vi "SaveP0(air).vi"(7 "error in (no error)":errorcluster, 10 "OSA Setting":T1={"CENTER(nm)"="850", "SPAN(nm)"="700", "RESOLUTION(nm)"="10", "SAMPLING(point)"="1001", "NEARBY AVG(point)"=50} {"NEARBY AVG(point)" min=0 max=300}) -> (0 "error out":errorcluster, 1 "Power":dbl[](array[numeric])=[0.0, 0.0, 0.0, 0.0, 0.0, 0.0, 0.0, 0.0, 0.0, 0.0, 0.0, 0.0, 0.0, 0.0, 0.0, 0.0, 0.0, 0.0, 0.0, 0.0, 0.0, 0.0, 0.0, 0.0, 0.0, 0.0, 0.0, 0.0, 0.0, 0.0, 0.0, 0.0, 0.0, 0.0, 0.0, 0.0, 0.0, 0.0, 0.0, 0.0, 0.0, 0.0, 0.0, 0.0, 0.0, 0.0, 0.0, 0.0, 0.0, 0.0, 0.0, 0.0, 0.0, 0.0, 0.0, 0.0, 0.0, 0.0, 0.0, 0.0, 0.0, 0.0, 0.0, 0.0, 0.0, 0.0, 0.0, 0.0, 0.0, 0.0, 0.0, 0.0, 0.0, 0.0, 0.0, 0.0, 0.0, 0.0, 0.0, 0.0, 0.0, 0.0, 0.0, 0.0, 0.0, 0.0, 0.0, 0.0, 0.0, 0.0, 0.0, 0.0, 0.0, 0.0, 0.0, 0.0, 0.0, 0.0, 0.0, 0.0, 0.0, 0.0, 0.0, 0.0, 0.0, 0.0, 0.0, 0.0, 0.0, 0.0, 0.0, 0.0, 0.0, 0.0, 0.0, 4.604e-06, 4.226e-06, 3.975e-06, 3.889e-06, 3.711e-06, 3.198e-06, 3.37e-06, 3.06e-06, 2.761e-06, 2.723e-06, 2.421e-06, 2.456e-06, 2.236e-06, 2.262e-06, 1.844e-06, 1.89e-06, 1.693e-06, 1.559e-06, 1.574e-06, 1.384e-06, 1.509e-06, 1.223e-06, 1.135e-06, 1.015e-06, 1.019e-06, 1.063e-06, 1.12e-06, 1.008e-06, 9.191e-07, 8.066e-07, 9.947e-07, 8.717e-07, 7.15e-07, 3.58e-07, 6.616e-07, 2.625e-07, 6.819e-07, 5.007e-07, 5.837e-07, 3.041e-07, 3.955e-07, 2.946e-07, 2.786e-07, 4.332e-07, 3.147e-07, 4.411e-07, 3.222e-07, 5.534e-07, 4.934e-07, 3.092e-07, 4.549e-07, 3.537e-07, 5.085e-07, 5.492e-07, 3.821e-07, 1.417e-07, 1.836e-07, 4.04e-07, 3.374e-07, 2.833e-07, 4.353e-07, 4.327e-07, 4.769e-07, 2.7e-07, 4.071e-07, 5.302e-07, 2.895e-07, 4.622e-07, 2.297e-07, 3.785e-07, 5.313e-07, 4.222e-07, 4.187e-07, 4.765e-07, 2.779e-07, 4.899e-07, 3.572e-07, 4.825e-07, 4.047e-07, 2.323e-07, 4.424e-07, 3.741e-07, 3.112e-07, 3.263e-07, 5.85e-07, 3.807e-07, 4.832e-07, 3.282e-07, 5.253e-07, 5.721e-07, 3.284e-07, 5.965e-07, 5.382e-07, 6.57e-07, 6.003e-07, 5.373e-07, 2.205e-07, 2.197e-07, 4.956e-07, 5.32e-07, 6.087e-07, 5.617e-07, 3.005e-07, 2.958e-07, 4.149e-07, 5.546e-07, 4.977e-07, 5.231e-07, 4.014e-07, 5.628e-07, 4.117e-07, 5.73e-07, 5.151e-07, 5.486e-07, 4.807e-07, 4.761e-07, 7.077e-07, 4.602e-07, 6.771e-07, 6.071e-07, 6.961e-07, 6.177e-07, 4.859e-07, 7.841e-07, 6.593e-07, 7.061e-07, 7.447e-07, 7.425e-07, 6.849e-07, 8.248e-07, 7.253e-07, 6.385e-07, 5.973e-07, 7.055e-07, 9.005e-07, 6.834e-07, 7.497e-07, 7.568e-07, 7.572e-07, 6.431e-07, 7.918e-07, 7.715e-07, 8.923e-07, 9.456e-07, 8.613e-07, 7.157e-07, 8.648e-07, 9.133e-07, 8.563e-07, 8.122e-07, 8.679e-07, 9.508e-07, 8.59e-07, 8.475e-07, 9.19e-07, 7.877e-07, 8.525e-07, 9.693e-07, 9.565e-07, 9.64e-07, 9.516e-07, 9.918e-07, 9.921e-07, 9.24e-07, 9.257e-07, 9.966e-07, 1.017e-06, 1.008e-06, 1.046e-06, 9.957e-07, 1.008e-06, 9.996e-07, 1.162e-06, 1.04e-06, 1.153e-06, 1.19e-06, 1.151e-06, 1.036e-06, 1.183e-06, 1.253e-06, 1.113e-06, 1.186e-06, 1.175e-06, 1.156e-06, 1.232e-06, 1.183e-06, 1.203e-06, 1.293e-06, 1.303e-06, 1.256e-06, 1.223e-06, 1.332e-06, 1.313e-06, 1.354e-06, 1.179e-06, 1.332e-06, 1.405e-06, 1.37e-06, 1.48e-06, 1.411e-06, 5.115e-06, 5.245e-06, 5.299e-06, 5.328e-06, 5.298e-06, 5.443e-06, 5.469e-06, 5.779e-06, 5.733e-06, 5.651e-06, 5.691e-06, 5.718e-06, 5.813e-06, 5.937e-06, 6.012e-06, 6e-06, 6.008e-06, 6.105e-06, 6.046e-06, 6.014e-06, 6.085e-06, 5.952e-06, 5.963e-06, 5.892e-06, 5.992e-06, 5.988e-06, 6.057e-06, 6.126e-06, 6.143e-06, 6.149e-06, 6.281e-06, 6.341e-06, 6.312e-06, 6.395e-06, 6.426e-06, 6.446e-06, 6.497e-06, 6.625e-06, 6.554e-06, 6.759e-06, 6.725e-06, 6.679e-06, 6.767e-06, 6.895e-06, 6.907e-06, 7.068e-06, 7.076e-06, 7.064e-06, 7.228e-06, 7.205e-06, 7.393e-06, 7.487e-06, 7.401e-06, 7.538e-06, 7.579e-06, 7.667e-06, 7.736e-06, 7.748e-06, 7.781e-06, 8.029e-06, 8.021e-06, 8.011e-06, 8.174e-06, 8.176e-06, 8.232e-06, 8.256e-06, 8.341e-06, 8.428e-06, 8.462e-06, 8.486e-06, 8.625e-06, 8.696e-06, 8.716e-06, 8.832e-06, 8.847e-06, 8.972e-06, 9.087e-06, 9.166e-06, 9.088e-06, 9.273e-06, 9.281e-06, 9.285e-06, 9.345e-06, 9.43e-06, 9.467e-06, 9.631e-06, 9.643e-06, 9.694e-06, 9.801e-06, 9.802e-06, 1e-05, 9.924e-06, 1.001e-05, 1.012e-05, 1.013e-05, 1.024e-05, 1.033e-05, 1.037e-05, 1.046e-05, 1.042e-05, 1.058e-05, 1.061e-05, 1.073e-05, 1.073e-05, 1.09e-05, 1.086e-05, 1.101e-05, 1.11e-05, 1.115e-05, 1.127e-05, 1.109e-05, 1.124e-05, 1.132e-05, 1.137e-05, 1.143e-05, 1.147e-05, 1.15e-05, 1.159e-05, 1.156e-05, 1.154e-05, 1.174e-05, 1.176e-05, 1.188e-05, 1.155e-05, 1.193e-05, 1.21e-05, 1.194e-05, 1.214e-05, 1.205e-05, 1.212e-05, 1.215e-05, 1.2e-05, 1.222e-05, 1.216e-05, 1.215e-05, 1.239e-05, 1.241e-05, 1.222e-05, 1.257e-05, 1.28e-05, 1.255e-05, 1.262e-05, 1.293e-05, 1.305e-05, 1.312e-05, 1.314e-05, 1.337e-05, 1.32e-05, 1.324e-05, 1.344e-05, 1.352e-05, 1.352e-05, 1.347e-05, 1.366e-05, 1.388e-05, 1.382e-05, 1.386e-05, 1.397e-05, 1.409e-05, 1.393e-05, 1.372e-05, 1.392e-05, 1.418e-05, 1.404e-05, 1.434e-05, 1.43e-05, 1.419e-05, 1.433e-05, 1.438e-05, 1.427e-05, 1.45e-05, 1.459e-05, 1.465e-05, 1.466e-05, 1.471e-05, 1.49e-05, 1.494e-05, 1.504e-05, 1.498e-05, 1.497e-05, 1.515e-05, 1.507e-05, 1.512e-05, 1.525e-05, 1.498e-05, 1.523e-05, 1.529e-05, 1.536e-05, 1.523e-05, 1.567e-05, 1.547e-05, 1.549e-05, 1.529e-05, 1.539e-05, 1.538e-05, 1.556e-05, 1.554e-05, 1.57e-05, 1.585e-05, 1.594e-05, 1.594e-05, 1.58e-05, 1.582e-05, 1.631e-05, 1.616e-05, 1.631e-05, 1.638e-05, 1.631e-05, 1.648e-05, 1.648e-05, 1.653e-05, 1.638e-05, 1.649e-05, 1.655e-05, 1.657e-05, 1.646e-05, 1.649e-05, 1.621e-05, 1.657e-05, 1.659e-05, 1.657e-05, 1.637e-05, 1.66e-05, 1.662e-05, 1.661e-05, 1.678e-05, 1.665e-05, 1.702e-05, 1.665e-05, 1.717e-05, 1.718e-05, 1.699e-05, 1.709e-05, 1.722e-05, 1.729e-05, 1.737e-05, 1.743e-05, 1.732e-05, 1.747e-05, 1.747e-05, 1.736e-05, 1.725e-05, 1.74e-05, 1.717e-05, 1.745e-05, 1.737e-05, 1.733e-05, 1.738e-05, 1.742e-05, 1.737e-05, 1.749e-05, 1.761e-05, 1.749e-05, 1.747e-05, 1.736e-05, 1.748e-05, 1.758e-05, 2.446e-05, 2.448e-05, 2.45e-05, 2.477e-05, 2.464e-05, 2.468e-05, 2.473e-05, 2.475e-05, 2.478e-05, 2.503e-05, 2.484e-05, 2.503e-05, 2.493e-05, 2.5e-05, 2.497e-05, 2.511e-05, 2.512e-05, 2.51e-05, 2.536e-05, 2.521e-05, 2.531e-05, 2.536e-05, 2.549e-05, 2.546e-05, 2.55e-05, 2.546e-05, 2.549e-05, 2.566e-05, 2.56e-05, 2.56e-05, 2.552e-05, 2.578e-05, 2.577e-05, 2.586e-05, 2.576e-05, 2.577e-05, 2.584e-05, 2.577e-05, 2.599e-05, 2.589e-05, 2.591e-05, 2.623e-05, 2.609e-05, 2.613e-05, 2.618e-05, 2.63e-05, 2.609e-05, 2.623e-05, 2.627e-05, 2.647e-05, 2.646e-05, 2.654e-05, 2.65e-05, 2.648e-05, 2.648e-05, 2.647e-05, 2.694e-05, 2.651e-05, 2.671e-05, 2.675e-05, 2.69e-05, 2.683e-05, 2.71e-05, 2.693e-05, 2.693e-05, 2.713e-05, 2.707e-05, 2.724e-05, 2.722e-05, 2.738e-05, 2.734e-05, 2.743e-05, 2.745e-05, 2.722e-05, 2.762e-05, 2.765e-05, 2.769e-05, 2.782e-05, 2.771e-05, 2.793e-05, 2.806e-05, 2.807e-05, 2.823e-05, 2.838e-05, 2.836e-05, 2.841e-05, 2.855e-05, 2.865e-05, 2.88e-05, 2.891e-05, 2.896e-05, 2.898e-05, 2.9e-05, 2.906e-05, 2.905e-05, 2.913e-05, 2.909e-05, 2.904e-05, 2.942e-05, 2.918e-05, 2.936e-05, 2.948e-05, 2.952e-05, 2.955e-05, 2.951e-05, 2.958e-05, 2.963e-05, 2.99e-05, 2.989e-05, 2.997e-05, 3.012e-05, 3.006e-05, 3.009e-05, 3.016e-05, 3.039e-05, 3.04e-05, 3.053e-05, 3.051e-05, 3.052e-05, 3.074e-05, 3.064e-05, 3.06e-05, 3.082e-05, 3.086e-05, 3.073e-05, 3.095e-05, 3.096e-05, 3.094e-05, 3.092e-05, 3.109e-05, 3.099e-05, 3.098e-05, 3.107e-05, 3.114e-05, 3.131e-05, 3.129e-05, 3.129e-05, 3.146e-05, 3.147e-05, 3.147e-05, 3.159e-05, 3.18e-05, 3.17e-05, 3.166e-05, 3.191e-05, 3.184e-05, 3.196e-05, 3.218e-05, 3.219e-05, 3.233e-05, 3.23e-05, 3.25e-05, 3.265e-05, 3.258e-05, 3.264e-05, 3.268e-05, 3.27e-05, 3.276e-05, 3.282e-05, 3.287e-05, 3.288e-05, 3.285e-05, 3.298e-05, 3.314e-05, 3.324e-05, 3.337e-05, 3.338e-05, 3.336e-05, 3.329e-05, 3.344e-05, 3.356e-05, 3.375e-05, 3.382e-05, 3.376e-05, 3.378e-05, 3.373e-05, 3.391e-05, 3.4e-05, 3.405e-05, 3.417e-05, 3.42e-05, 3.443e-05, 3.431e-05, 3.435e-05, 3.445e-05, 3.431e-05, 3.446e-05, 3.448e-05, 3.449e-05, 3.467e-05, 3.455e-05, 3.47e-05, 3.483e-05, 3.498e-05, 3.476e-05, 3.492e-05, 3.492e-05, 3.502e-05, 3.515e-05, 3.522e-05, 3.538e-05, 3.537e-05, 3.537e-05, 3.553e-05, 3.55e-05, 3.56e-05, 3.57e-05, 3.583e-05, 3.578e-05, 3.592e-05, 3.603e-05, 3.601e-05, 3.605e-05, 3.61e-05, 3.615e-05, 3.627e-05, 3.638e-05, 3.621e-05, 3.619e-05, 3.639e-05, 3.632e-05, 3.651e-05, 3.647e-05, 3.671e-05, 3.668e-05, 3.675e-05, 3.66e-05, 3.677e-05, 3.664e-05, 3.686e-05, 3.655e-05, 3.676e-05, 3.666e-05, 3.667e-05, 3.667e-05, 3.661e-05, 3.66e-05, 3.674e-05, 3.673e-05, 3.659e-05, 3.68e-05, 3.678e-05, 3.684e-05, 3.678e-05, 3.672e-05, 3.669e-05, 3.672e-05, 3.664e-05, 3.661e-05, 3.665e-05, 3.68e-05, 3.669e-05, 3.679e-05, 3.678e-05, 3.713e-05, 3.693e-05, 3.724e-05, 3.724e-05, 3.73e-05, 3.738e-05, 3.742e-05, 3.764e-05, 3.771e-05, 3.766e-05, 3.786e-05, 3.787e-05, 3.778e-05, 3.779e-05, 3.771e-05, 3.767e-05, 3.755e-05, 3.742e-05, 3.749e-05, 3.756e-05, 3.756e-05, 3.759e-05, 3.748e-05, 3.769e-05, 3.778e-05, 3.785e-05, 3.787e-05, 3.812e-05, 3.799e-05, 3.811e-05, 3.822e-05, 3.832e-05, 3.828e-05, 3.838e-05, 3.87e-05, 3.863e-05, 3.879e-05, 3.871e-05, 3.877e-05, 3.883e-05, 3.872e-05, 3.891e-05, 3.877e-05, 3.9e-05, 3.898e-05, 3.905e-05, 3.885e-05, 3.892e-05, 3.89e-05, 3.901e-05, 3.879e-05, 3.89e-05, 3.885e-05, 3.891e-05, 3.895e-05, 3.89e-05, 3.891e-05, 3.883e-05, 3.875e-05, 3.872e-05, 3.896e-05, 3.883e-05, 3.888e-05, 3.9e-05, 3.899e-05, 3.914e-05, 3.913e-05, 3.923e-05, 3.929e-05, 3.932e-05, 3.936e-05, 3.914e-05, 3.924e-05, 3.95e-05, 3.932e-05, 3.929e-05, 3.931e-05, 3.938e-05, 3.918e-05, 3.9280000000000003e-05, 3.925e-05, 3.936e-05, 3.947e-05, 3.912e-05, 3.931e-05, 3.945e-05, 3.94e-05, 3.941e-05, 3.94e-05, 3.913e-05, 3.903e-05, 3.915e-05, 3.908e-05, 3.912e-05, 3.903e-05, 3.89e-05, 3.898e-05, 3.885e-05, 3.881e-05, 3.883e-05, 3.879e-05, 3.886e-05, 3.904e-05, 3.903e-05, 3.891e-05, 3.871e-05, 3.868e-05, 3.847e-05, 3.858e-05, 3.857e-05, 3.846e-05, 3.852e-05, 3.857e-05, 3.871e-05, 3.873e-05, 3.859e-05, 3.87e-05, 3.88e-05, 3.862e-05, 3.851e-05, 3.855e-05, 3.837e-05, 3.839e-05, 3.831e-05, 3.84e-05, 3.833e-05, 3.844e-05, 3.835e-05, 3.838e-05, 3.837e-05, 3.84e-05, 3.845e-05, 3.835e-05, 3.841e-05, 3.82e-05, 3.82e-05, 3.805e-05, 3.808e-05, 3.801e-05, 3.788e-05, 3.796e-05, 3.797e-05, 3.778e-05, 3.795e-05, 3.768e-05, 3.771e-05, 3.783e-05, 3.767e-05, 3.754e-05, 3.754e-05, 3.761e-05, 3.76e-05, 3.774e-05, 3.765e-05, 3.757e-05, 3.777e-05, 3.755e-05, 3.753e-05, 3.754e-05, 3.758e-05, 3.758e-05, 3.771e-05, 3.766e-05, 3.766e-05, 3.781e-05, 3.785e-05, 3.791e-05, 3.799e-05, 3.795e-05, 3.794e-05, 3.808e-05, 3.79e-05, 3.809e-05, 3.798e-05, 3.794e-05], 3 "Wavelength":dbl[](array[numeric])=[250.0, 250.7, 251.4, 252.1, 252.8, 253.5, 254.2, 254.9, 255.6, 256.3, 257.0, 257.7, 258.4, 259.1, 259.8, 260.5, 261.2, 261.9, 262.6, 263.3, 264.0, 264.7, 265.4, 266.1, 266.8, 267.5, 268.2, 268.9, 269.6, 270.3, 271.0, 271.7, 272.4, 273.1, 273.8, 274.5, 275.2, 275.9, 276.6, 277.3, 278.0, 278.7, 279.4, 280.1, 280.8, 281.5, 282.2, 282.9, 283.6, 284.3, 285.0, 285.7, 286.4, 287.1, 287.8, 288.5, 289.2, 289.9, 290.6, 291.3, 292.0, 292.7, 293.4, 294.1, 294.8, 295.5, 296.2, 296.9, 297.6, 298.3, 299.0, 299.7, 300.4, 301.1, 301.8, 302.5, 303.2, 303.9, 304.6, 305.3, 306.0, 306.7, 307.4, 308.1, 308.8, 309.5, 310.2, 310.9, 311.6, 312.3, 313.0, 313.7, 314.4, 315.1, 315.8, 316.5, 317.2, 317.9, 318.6, 319.3, 320.0, 320.7, 321.4, 322.1, 322.8, 323.5, 324.2, 324.9, 325.6, 326.3, 327.0, 327.7, 328.4, 329.1, 329.8, 330.5, 331.2, 331.9, 332.6, 333.3, 334.0, 334.7, 335.4, 336.1, 336.8, 337.5, 338.2, 338.9, 339.6, 340.3, 341.0, 341.7, 342.4, 343.1, 343.8, 344.5, 345.2, 345.9, 346.6, 347.3, 348.0, 348.7, 349.4, 350.1, 350.8, 351.5, 352.2, 352.9, 353.6, 354.3, 355.0, 355.7, 356.4, 357.1, 357.8, 358.5, 359.2, 359.9, 360.6, 361.3, 362.0, 362.7, 363.4, 364.1, 364.8, 365.5, 366.2, 366.9, 367.6, 368.3, 369.0, 369.7, 370.4, 371.1, 371.8, 372.5, 373.2, 373.9, 374.6, 375.3, 376.0, 376.7, 377.4, 378.1, 378.8, 379.5, 380.2, 380.9, 381.6, 382.3, 383.0, 383.7, 384.4, 385.1, 385.8, 386.5, 387.2, 387.9, 388.6, 389.3, 390.0, 390.7, 391.4, 392.1, 392.8, 393.5, 394.2, 394.9, 395.6, 396.3, 397.0, 397.7, 398.4, 399.1, 399.8, 400.5, 401.2, 401.9, 402.6, 403.3, 404.0, 404.7, 405.4, 406.1, 406.8, 407.5, 408.2, 408.9, 409.6, 410.3, 411.0, 411.7, 412.4, 413.1, 413.8, 414.5, 415.2, 415.9, 416.6, 417.3, 418.0, 418.7, 419.4, 420.1, 420.8, 421.5, 422.2, 422.9, 423.6, 424.3, 425.0, 425.7, 426.4, 427.1, 427.8, 428.5, 429.2, 429.9, 430.6, 431.3, 432.0, 432.7, 433.4, 434.1, 434.8, 435.5, 436.2, 436.9, 437.6, 438.3, 439.0, 439.7, 440.4, 441.1, 441.8, 442.5, 443.2, 443.9, 444.6, 445.3, 446.0, 446.7, 447.4, 448.1, 448.8, 449.5, 450.2, 450.9, 451.6, 452.3, 453.0, 453.7, 454.4, 455.1, 455.8, 456.5, 457.2, 457.9, 458.6, 459.3, 460.0, 460.7, 461.4, 462.1, 462.8, 463.5, 464.2, 464.9, 465.6, 466.3, 467.0, 467.7, 468.4, 469.1, 469.8, 470.5, 471.2, 471.9, 472.6, 473.3, 474.0, 474.7, 475.4, 476.1, 476.8, 477.5, 478.2, 478.9, 479.6, 480.3, 481.0, 481.7, 482.4, 483.1, 483.8, 484.5, 485.2, 485.9, 486.6, 487.3, 488.0, 488.7, 489.4, 490.1, 490.8, 491.5, 492.2, 492.9, 493.6, 494.3, 495.0, 495.7, 496.4, 497.1, 497.8, 498.5, 499.2, 499.9, 500.6, 501.3, 502.0, 502.7, 503.4, 504.1, 504.8, 505.5, 506.2, 506.9, 507.6, 508.3, 509.0, 509.7, 510.4, 511.1, 511.8, 512.5, 513.2, 513.9, 514.6, 515.3, 516.0, 516.7, 517.4, 518.1, 518.8, 519.5, 520.2, 520.9, 521.6, 522.3, 523.0, 523.7, 524.4, 525.1, 525.8, 526.5, 527.2, 527.9, 528.6, 529.3, 530.0, 530.7, 531.4, 532.1, 532.8, 533.5, 534.2, 534.9, 535.6, 536.3, 537.0, 537.7, 538.4, 539.1, 539.8, 540.5, 541.2, 541.9, 542.6, 543.3, 544.0, 544.7, 545.4, 546.1, 546.8, 547.5, 548.2, 548.9, 549.6, 550.3, 551.0, 551.7, 552.4, 553.1, 553.8, 554.5, 555.2, 555.9, 556.6, 557.3, 558.0, 558.7, 559.4, 560.1, 560.8, 561.5, 562.2, 562.9, 563.6, 564.3, 565.0, 565.7, 566.4, 567.1, 567.8, 568.5, 569.2, 569.9, 570.6, 571.3, 572.0, 572.7, 573.4, 574.1, 574.8, 575.5, 576.2, 576.9, 577.6, 578.3, 579.0, 579.7, 580.4, 581.1, 581.8, 582.5, 583.2, 583.9, 584.6, 585.3, 586.0, 586.7, 587.4, 588.1, 588.8, 589.5, 590.2, 590.9, 591.6, 592.3, 593.0, 593.7, 594.4, 595.1, 595.8, 596.5, 597.2, 597.9, 598.6, 599.3, 600.0, 600.7, 601.4, 602.1, 602.8, 603.5, 604.2, 604.9, 605.6, 606.3, 607.0, 607.7, 608.4, 609.1, 609.8, 610.5, 611.2, 611.9, 612.6, 613.3, 614.0, 614.7, 615.4, 616.1, 616.8, 617.5, 618.2, 618.9, 619.6, 620.3, 621.0, 621.7, 622.4, 623.1, 623.8, 624.5, 625.2, 625.9, 626.6, 627.3, 628.0, 628.7, 629.4, 630.1, 630.8, 631.5, 632.2, 632.9, 633.6, 634.3, 635.0, 635.7, 636.4, 637.1, 637.8, 638.5, 639.2, 639.9, 640.6, 641.3, 642.0, 642.7, 643.4, 644.1, 644.8, 645.5, 646.2, 646.9, 647.6, 648.3, 649.0, 649.7, 650.4, 651.1, 651.8, 652.5, 653.2, 653.9, 654.6, 655.3, 656.0, 656.7, 657.4, 658.1, 658.8, 659.5, 660.2, 660.9, 661.6, 662.3, 663.0, 663.7, 664.4, 665.1, 665.8, 666.5, 667.2, 667.9, 668.6, 669.3, 670.0, 670.7, 671.4, 672.1, 672.8, 673.5, 674.2, 674.9, 675.6, 676.3, 677.0, 677.7, 678.4, 679.1, 679.8, 680.5, 681.2, 681.9, 682.6, 683.3, 684.0, 684.7, 685.4, 686.1, 686.8, 687.5, 688.2, 688.9, 689.6, 690.3, 691.0, 691.7, 692.4, 693.1, 693.8, 694.5, 695.2, 695.9, 696.6, 697.3, 698.0, 698.7, 699.4, 700.1, 700.8, 701.5, 702.2, 702.9, 703.6, 704.3, 705.0, 705.7, 706.4, 707.1, 707.8, 708.5, 709.2, 709.9, 710.6, 711.3, 712.0, 712.7, 713.4, 714.1, 714.8, 715.5, 716.2, 716.9, 717.6, 718.3, 719.0, 719.7, 720.4, 721.1, 721.8, 722.5, 723.2, 723.9, 724.6, 725.3, 726.0, 726.7, 727.4, 728.1, 728.8, 729.5, 730.2, 730.9, 731.6, 732.3, 733.0, 733.7, 734.4, 735.1, 735.8, 736.5, 737.2, 737.9, 738.6, 739.3, 740.0, 740.7, 741.4, 742.1, 742.8, 743.5, 744.2, 744.9, 745.6, 746.3, 747.0, 747.7, 748.4, 749.1, 749.8, 750.5, 751.2, 751.9, 752.6, 753.3, 754.0, 754.7, 755.4, 756.1, 756.8, 757.5, 758.2, 758.9, 759.6, 760.3, 761.0, 761.7, 762.4, 763.1, 763.8, 764.5, 765.2, 765.9, 766.6, 767.3, 768.0, 768.7, 769.4, 770.1, 770.8, 771.5, 772.2, 772.9, 773.6, 774.3, 775.0, 775.7, 776.4, 777.1, 777.8, 778.5, 779.2, 779.9, 780.6, 781.3, 782.0, 782.7, 783.4, 784.1, 784.8, 785.5, 786.2, 786.9, 787.6, 788.3, 789.0, 789.7, 790.4, 791.1, 791.8, 792.5, 793.2, 793.9, 794.6, 795.3, 796.0, 796.7, 797.4, 798.1, 798.8, 799.5, 800.2, 800.9, 801.6, 802.3, 803.0, 803.7, 804.4, 805.1, 805.8, 806.5, 807.2, 807.9, 808.6, 809.3, 810.0, 810.7, 811.4, 812.1, 812.8, 813.5, 814.2, 814.9, 815.6, 816.3, 817.0, 817.7, 818.4, 819.1, 819.8, 820.5, 821.2, 821.9, 822.6, 823.3, 824.0, 824.7, 825.4, 826.1, 826.8, 827.5, 828.2, 828.9, 829.6, 830.3, 831.0, 831.7, 832.4, 833.1, 833.8, 834.5, 835.2, 835.9, 836.6, 837.3, 838.0, 838.7, 839.4, 840.1, 840.8, 841.5, 842.2, 842.9, 843.6, 844.3, 845.0, 845.7, 846.4, 847.1, 847.8, 848.5, 849.2, 849.9, 850.6, 851.3, 852.0, 852.7, 853.4, 854.1, 854.8, 855.5, 856.2, 856.9, 857.6, 858.3, 859.0, 859.7, 860.4, 861.1, 861.8, 862.5, 863.2, 863.9, 864.6, 865.3, 866.0, 866.7, 867.4, 868.1, 868.8, 869.5, 870.2, 870.9, 871.6, 872.3, 873.0, 873.7, 874.4, 875.1, 875.8, 876.5, 877.2, 877.9, 878.6, 879.3, 880.0, 880.7, 881.4, 882.1, 882.8, 883.5, 884.2, 884.9, 885.6, 886.3, 887.0, 887.7, 888.4, 889.1, 889.8, 890.5, 891.2, 891.9, 892.6, 893.3, 894.0, 894.7, 895.4, 896.1, 896.8, 897.5, 898.2, 898.9, 899.6, 900.3, 901.0, 901.7, 902.4, 903.1, 903.8, 904.5, 905.2, 905.9, 906.6, 907.3, 908.0, 908.7, 909.4, 910.1, 910.8, 911.5, 912.2, 912.9, 913.6, 914.3, 915.0, 915.7, 916.4, 917.1, 917.8, 918.5, 919.2, 919.9, 920.6, 921.3, 922.0, 922.7, 923.4, 924.1, 924.8, 925.5, 926.2, 926.9, 927.6, 928.3, 929.0, 929.7, 930.4, 931.1, 931.8, 932.5, 933.2, 933.9, 934.6, 935.3, 936.0, 936.7, 937.4, 938.1, 938.8, 939.5, 940.2, 940.9, 941.6, 942.3, 943.0, 943.7, 944.4, 945.1, 945.8, 946.5, 947.2, 947.9, 948.6, 949.3, 950.0])   [LabVIEW 2020]
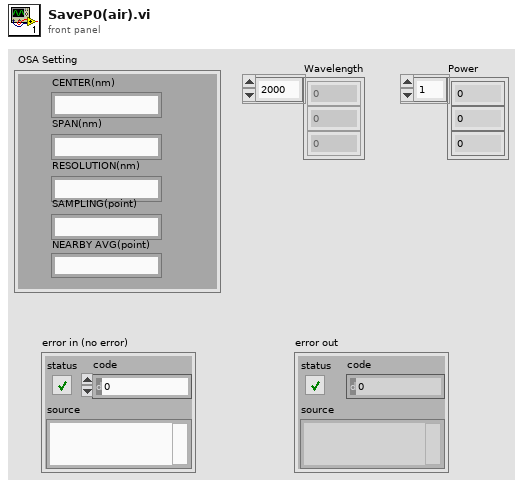
[diagram p1: front panel]
types:
  T1 = cluster{"CENTER(nm)":string, "SPAN(nm)":string, "RESOLUTION(nm)":string, "SAMPLING(point)":string, "NEARBY AVG(point)":i32}
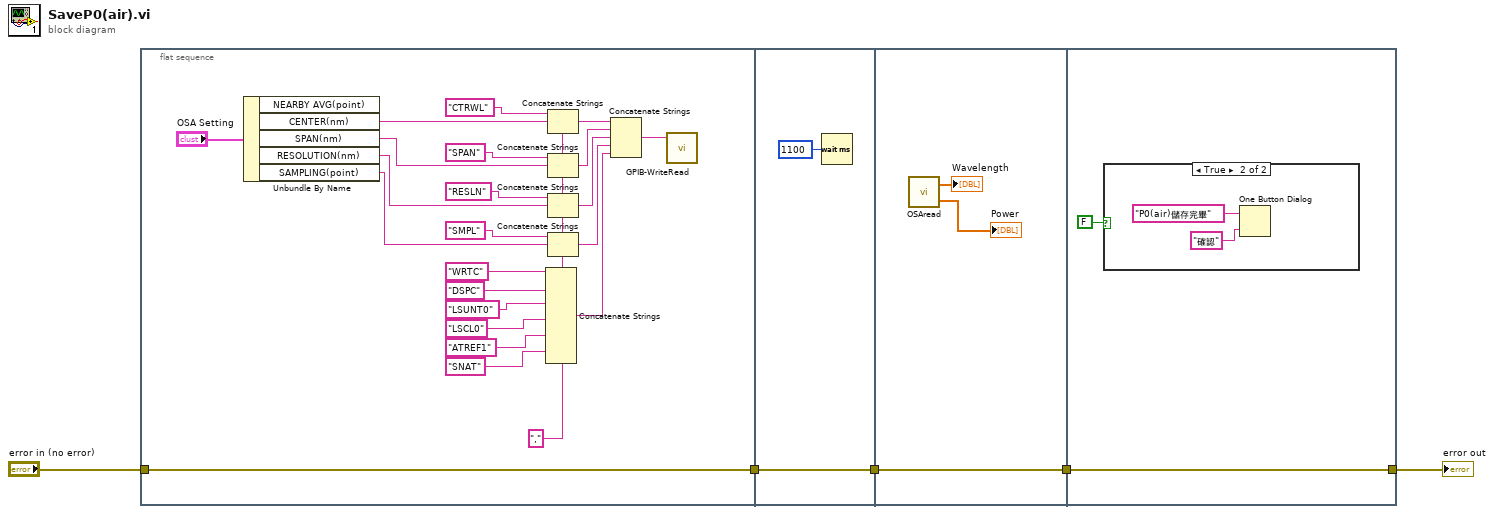
[diagram p0: block diagram]
diagram:
  n1 = flat-sequence {
    tunnel: [w6] -> w5
    tunnel: "error in (no error)" -> [w6]
    tunnel: w5 -> [w29]
    tunnel: [w29] -> w2
    tunnel: [w32] -> w3
    tunnel: w2 -> [w32]
    tunnel: w3 -> [w34]
    tunnel: [w34] -> w1
    frame #0 {
      w16 = ","
      n2 = Unbundle By Name("OSA Setting") -> ("CENTER(nm)"=w28:string, "SPAN(nm)"=w27:string, "RESOLUTION(nm)"=w26:string, "SAMPLING(point)"=w25:string)  [unwired: 1 out]
      n3 = Concatenate Strings("WRTC", w16, "DSPC", w16, "LSUNT0", w16, "LSCL0", w16, "ATREF1", w16, "SNAT", w16) -> (w19:string)
      n4 = Concatenate Strings("CTRWL", w28, w16) -> (w23:string)
      n5 = Concatenate Strings("SPAN", w27, w16) -> (w22:string)
      n6 = Concatenate Strings("RESLN", w26, w16) -> (w21:string)
      n7 = Concatenate Strings("SMPL", w25, w16) -> (w20:string)
      n8 = Concatenate Strings(w23, w22, w21, w20, w19) -> (w18:string)
      n9 = call "GPIB-WriteRead.vi"("Characters to Write"=w18) -> ()  [unwired: 1 in, 3 out]
    }
    frame #1 {
      n10 = Wait (ms)(milliseconds to wait=u32 1100) -> ()  [unwired: 1 out]
    }
    frame #2 {
      n11 = call "OSAread.vi"() -> ("power"=→"Power":dbl[], "length"=→"Wavelength":dbl[])  [unwired: 2 out]
    }
    frame #3 {
      n12 = case shown="True" FALSE {
        frame False {
        }
        frame True {
          n13 = One Button Dialog(message="P0(air)儲存完畢", button name ("OK")="確認") -> ()  [unwired: 1 out]
        }
      }
    }
  }
  "error out" <- w1
